vi "Check_Traverse_move_Low.vi"(3 "Traverse Name":string, 4 "Rotation (deg)":dbl format="%#.2f", 5 "Exclude Array":T1[](array[typedef])=[{"Sizes"=[{"Max"=15000.0, "Min"=0.0}, {"Max"=1000.0, "Min"=-1000.0}, {"Max"=300.0, "Min"=0.0}], "Name"="Roughness Elements", "Exclude Type"=enum."Allow only vertical moves"}, {"Sizes"=[{"Max"=17000.0, "Min"=16000.0}, {"Max"=200.0, "Min"=-200.0}, {"Max"=-50.0, "Min"=-250.0}], "Name"="B204", "Exclude Type"=enum."Exclude completely"}] {"Sizes"."Min" format="%#.1f"; "Sizes"."Max" format="%#.1f"}, 7 "Probe Volume":T2=[{"Max"=15.0, "Min"=-15.0}, {"Max"=250.0, "Min"=0.0}, {"Max"=15.0, "Min"=-15.0}] {"Min" format="%#.1f"; "Max" format="%#.1f"}, 8 "New Position":dbl[](array[numeric])=[0.0, 0.0, 0.0] format="%.2f", 9 "Current position":dbl[](array[numeric])=[0.0, 0.0, 0.0] format="%.2f") -> (0 "Error Comments":string, 2 "Position At Crash":dbl[](array[numeric]) format="%.2f")   [LabVIEW 2010]
uses:
  Box_size.ctl
  Exclude_cluster.ctl
  Exclusion_type.ctl
panel:
  out "Numeric":i32
  # "X                Y                   Z"
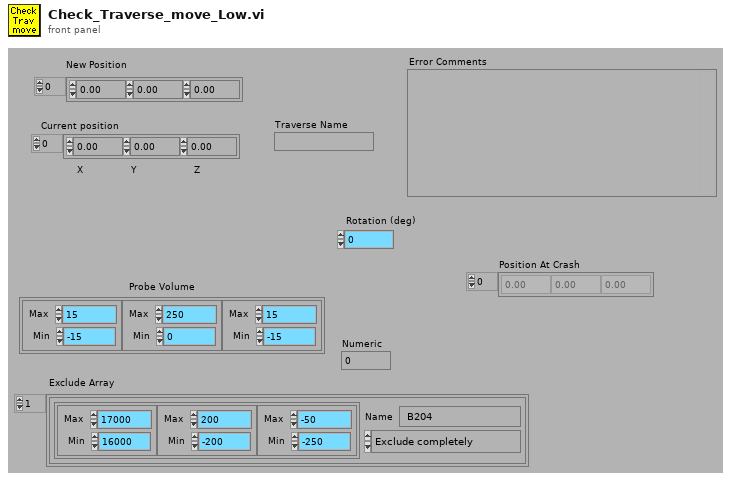
[diagram p1: front panel]
types:
  T1 = typedef "Exclude_cluster.ctl" = cluster{"Sizes":T2, "Name":string, "Exclude Type":T3}
  T2 = typedef "Box_size.ctl" = cluster{"Max":dbl, "Min":dbl}[]
  T3 = typedef "Exclusion_type.ctl" = enum16{"Exclude completely", "Allow only vertical moves"}
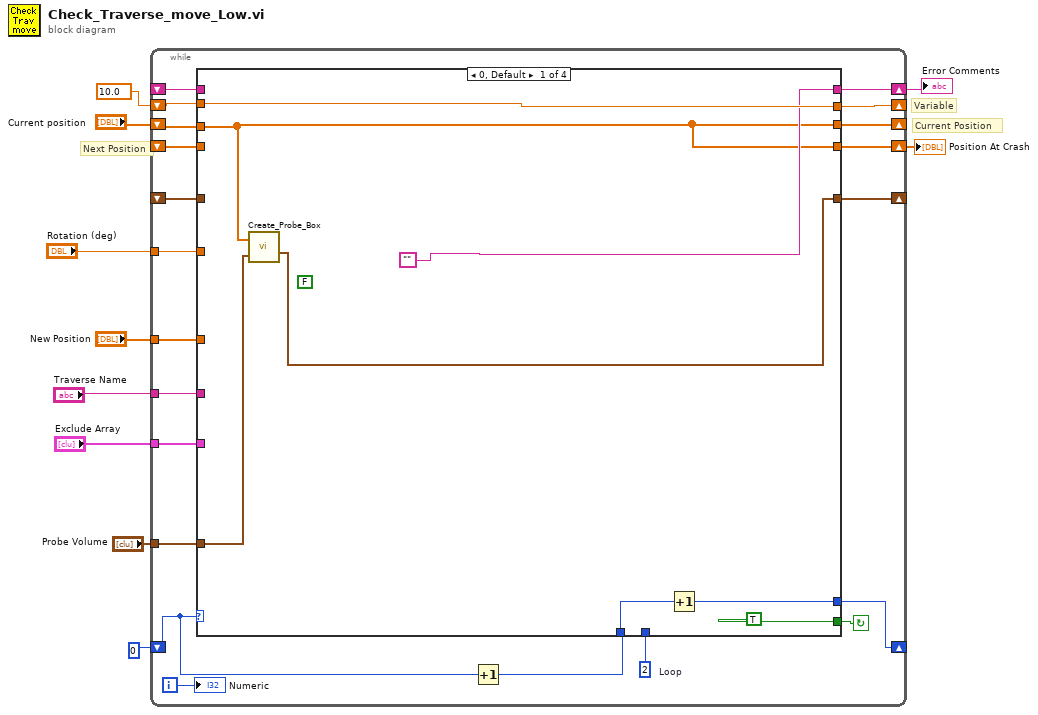
[diagram p0: block diagram]
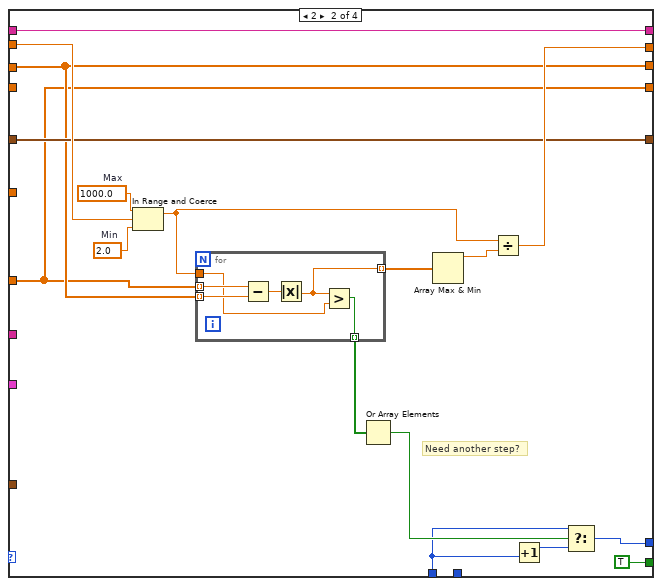
[diagram p2: hidden frame]
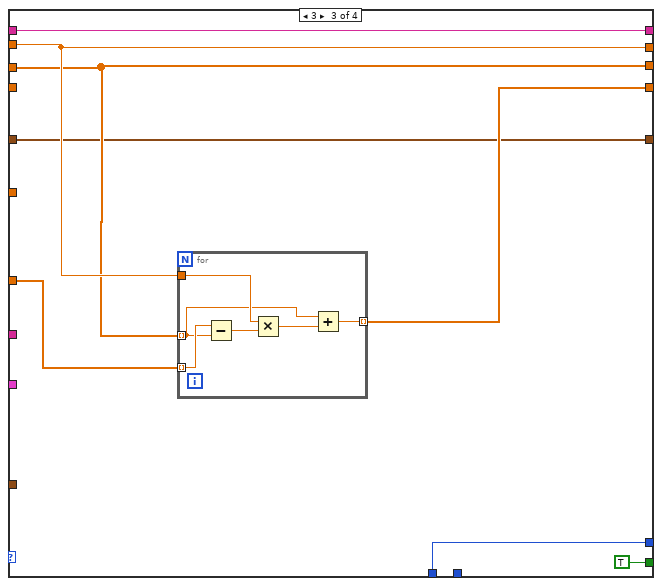
[diagram p3: hidden frame]
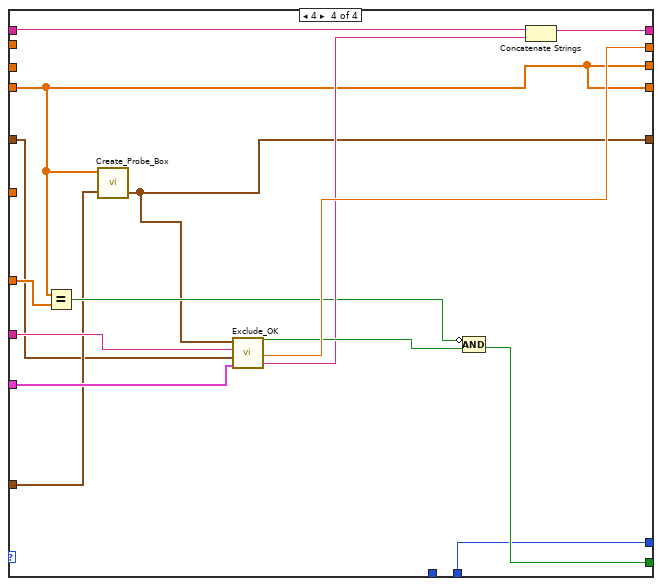
[diagram p4: hidden frame]
diagram:
  # "Current Position"
  # "Next Position"
  # "Variable"
  n1 = while {
    shift-left: _ -> [w12]
    shift-right: [w13] -> _
    tunnel: "Probe Volume" -> [w15]
    tunnel: "New Position" -> [w17]
    shift-left: _ -> [w19]
    shift-right: [w20] -> w6
    shift-left: 0 -> [w23]
    shift-right: [w22] -> _
    tunnel: "Traverse Name" -> [w24]
    tunnel: "Exclude Array" -> [w26]
    shift-left: 10.0 ("Separation Distance") -> [w30]
    shift-right: [w25] -> _
    shift-left: _ -> [w18]
    shift-right: [w28] -> w4
    shift-left: "Current position" -> [w31]
    shift-right: [w29] -> _
    tunnel: "Rotation (deg)" -> [w11]
    i -> [w14]
    stop <- w27 continue-if-true
    w16 = 2  # Loop
    n2 = Increment(x=w23) -> (x+1=w21:i32)
    n3 = case shown="0, Default" w23 {
      tunnel: w31 -> [w33 w42 w67 _]
      tunnel: w30 -> [w39 w56 w68 _]
      tunnel: [w33 w42 w67 w82] -> w29
      tunnel: [w33 w41 w66 w82] -> w28
      tunnel: [TRUE ("Box Inside") TRUE ("Box Inside") TRUE ("Box Inside") w80] -> w27
      tunnel: w15 -> [w37 _ _ w81]
      tunnel: w26 -> [_ _ _ w91]
      tunnel: [w39 w48 w68 w90] -> w25
      tunnel: w24 -> [_ _ _ w89]
      tunnel: [w32 w46 w64 w79] -> w22
      tunnel: w21 -> [w36 w44 w64 _]
      tunnel: ["" w54 w70 w86] -> w20
      tunnel: w19 -> [_ w54 w70 w87]
      tunnel: w18 -> [_ _ _ w82]
      tunnel: w17 -> [_ w41 w65 w84]
      tunnel: w16 -> [_ _ _ w79]
      tunnel: [w34 w43 w63 w78] -> w13
      tunnel: w12 -> [_ w43 w63 w77]
      tunnel: w11 -> [_ _ _ _]
      frame 0, Default {
        (unwired) FALSE
        n4 = call "Create_Probe_Box.vi"("Probe Volume"=w37, "Probe Position"=w33) -> ("Current Probe Volume"=w34:cluster{"Max":dbl, "Min":dbl}[])
        n5 = Increment(x=w36) -> (x+1=w32:i32)
      }
      frame 2 {
        w51 = 1000.0  # Max
        w52 = 2.0  # Min
        # "Need another step?"
        n6 = In Range and Coerce(upper limit=w51, x=w56, lower limit=w52) -> (coerced(x)=w40:dbl)  [unwired: 1 out]
        n7 = for {
          tunnel: w41 -> [w62] mode=indexing
          tunnel: w42 -> [w61] mode=indexing
          tunnel: w40 -> [w60]
          tunnel: [w58] -> w53 mode=indexing
          tunnel: [w57] -> w50 mode=indexing
          n8 = Subtract(x=w62, y=w61) -> (x-y=w59:dbl)
          n9 = Absolute Value(x=w59) -> (abs(x)=w57:dbl)
          n10 = Greater?(x=w57, y=w60) -> (0:w58:bool)
        }
        n11 = Or Array Elements(Boolean array=w53) -> (logical OR=w47:bool)
        n12 = Array Max & Min(array=w50) -> (max value=w49:dbl)  [unwired: 3 out]
        n13 = Divide(x=w40, y=w49) -> (x/y=w48:dbl)
        n14 = Increment(x=w44) -> (x+1=w45:i32)
        n15 = Select(t=w44, s=w47, f=w45) -> (s? t:f=w46:i32)
      }
      frame 3 {
        n16 = for {
          tunnel: w65 -> [w76] mode=indexing
          tunnel: w67 -> [w72] mode=indexing
          tunnel: w68 -> [w74]
          tunnel: [w71] -> w66 mode=indexing
          n17 = Subtract(x=w76, y=w72) -> (x-y=w75:dbl)
          n18 = Multiply(x=w74, y=w75) -> (x*y=w73:dbl)
          n19 = Add(x=w72, y=w73) -> (x+y=w71:dbl)
        }
      }
      frame 4 {
        n20 = Equal?(x=w82, y=w84) -> (x = y?=w83:bool)
        n21 = call "Create_Probe_Box.vi"("Probe Volume"=w81, "Probe Position"=w82) -> ("Current Probe Volume"=w78:cluster{"Max":dbl, "Min":dbl}[])
        n22 = call "Exclude_OK.vi"("Exclude Array"=w91, "Previous Probe Volume"=w77, "Traverse Name"=w89, "Probe Volume"=w78) -> ("Error Comments"=w85:string, "Separation Distance"=w90:dbl, "Probe OK?"=w88:bool)
        n23 = Compound Arithmetic op=AND(invert w83, w88) -> (w80:bool)
        n24 = Concatenate Strings(w87, w85) -> (w86:string)
      }
    }
    "Numeric" <- w14
  }
  "Error Comments" <- w6
  "Position At Crash" <- w4
